vi "ritter profile.vi"(8 "error in (no error)":errorcluster, 11 "VISA in":refnum<visa-resource-name>) -> (0 "error out":errorcluster, 2 "profile":string, 3 "VISA out":refnum<visa-resource-name>)   [LabVIEW 2020]
doc: "This vi returns the current profile of the Ritter gasmeter, which includes the Type and Power Status."
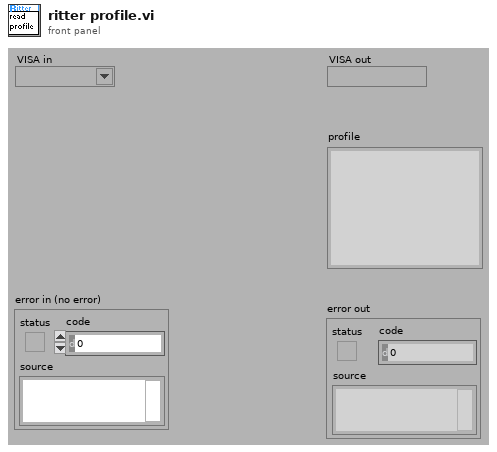
[diagram p1: front panel]
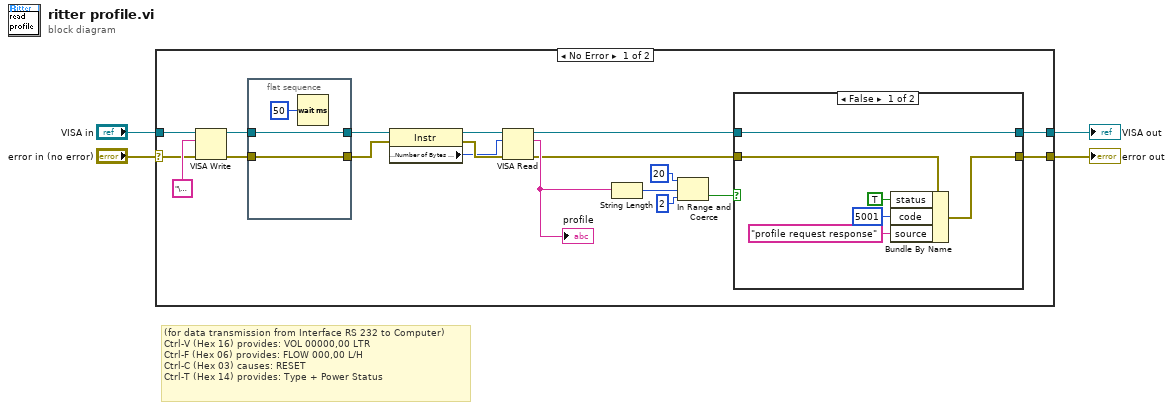
[diagram p0: block diagram]
diagram:
  # "(for data transmission from Interface RS 232 to Computer)\nCtrl-V (Hex 16) provides: VOL 00000,00 LTR\nCtrl-F (Hex 06) provides: FLOW 000,00 L/H\nCtrl-C (Hex 03) causes: RESET\nCtrl-T (Hex 14) provides: Type + Power Status"
  n1 = case shown="No Error" "error in (no error)" {
    selector: "error in (no error)" -> [w14 w35]
    tunnel: [w7 w35] -> w4
    tunnel: "VISA in" -> [w15 w36]
    tunnel: [w5 w36] -> w2
    frame No Error {
      n2 = VISA Write(VISA resource name=w15, write buffer="\u0014" ("string"), error in (no error)=w14) -> (VISA resource name out=w21:refnum<visa-resource-name>, error out=w22:errorcluster)  [unwired: 1 out]
      n3 = flat-sequence {
        tunnel: w22 -> [w34]
        tunnel: [w34] -> w20
        tunnel: w21 -> [w33]
        tunnel: [w33] -> w19
        frame #0 {
          n4 = Wait (ms)(milliseconds to wait=u32 50) -> ()  [unwired: 1 out]
        }
      }
      n5 = property class="Instr"(reference=w19, error in=w20) -> (reference out=w18:refnum<visa-resource-name>, error out=w17:errorcluster, "Serial Settings:Number of Bytes at Serial Port"=w16:u32)
      n6 = VISA Read(VISA resource name=w18, byte count=w16, error in (no error)=w17) -> (VISA resource name out=w6:refnum<visa-resource-name>, read buffer=w13:string, error out=w8:errorcluster)  [unwired: 1 out]
      "profile" <- w13
      n7 = String Length(string=w13) -> (length=w12:i32)
      n8 = In Range and Coerce(upper limit=20, x=w12, lower limit=2) -> (In Range?=w9:bool)  [unwired: 1 out]
      n9 = case shown="False" w9 {
        tunnel: w8 -> [w25 w31]
        tunnel: [w24 w31] -> w7
        tunnel: w6 -> [w29 w30]
        tunnel: [w29 w30] -> w5
        frame False {
          n10 = Bundle By Name(cluster=w25, "status"=TRUE, "code"=5001, "source"="profile request response") -> (w24:errorcluster)
        }
        frame True {
        }
      }
    }
    frame Error {
    }
  }
  "error out" <- w4
  "VISA out" <- w2
